vi "Robot Main.vi"() -> ()   [LabVIEW 2015]
doc: "This VI implements the framework and scheduler for your robotics program. It should not be necessary to modify the framework. You are expected to add your code to the VIs called from Robot Main - the ones located in the Team Code folder within the project."
uses:
  <vilib>/Rock Robotics/WPI/Camera/WPI_CameraImageSize.ctl
  <vilib>/Rock Robotics/WPI/Relay/WPI_RelayValue.ctl
  Robot Global Data.vi
  <vilib>/Rock Robotics/WPI/Utilities/WPI_GetSetVariantRefNum.vi
  <vilib>/Rock Robotics/WPI/Solenoid/Deprecated/WPI_SolenoidSetBool.vi
panel:
  in  "Image Size":T1=enum."320x240"
  in  "Enable Vision":bool
  in  "Finish":bool
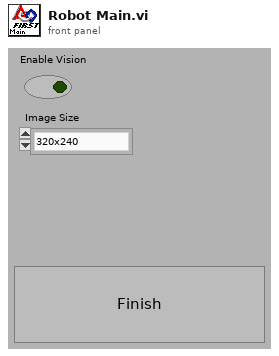
[diagram p1: front panel]
types:
  T1 = typedef "WPI_CameraImageSize.ctl" = enum16{"640x480", "320x240", "160x120", "Custom"}
  T2 = typedef "WPI_RelayValue.ctl" = enum16{"Off", "On", "Forward", "Reverse"}
  T3 = typedef "WPI_DriverStationDerivedRobotMode.ctl" = enum16{"Init", "Execute", "Stop"}
  T4 = typedef "WPI_DriverStationRobotMode2.ctl" = enum16{"Autonomous Disabled", "Autonomous Enabled", "Teleop Disabled", "Teleop Enabled", "Disconnected", "Finish", "Test Disabled", "Test Enabled", "Emergency Stopped"}
  T5 = typedef "WPI_JoystickDevRef.ctl" = cluster{"Device":T6}
  T6 = typedef "WPI_JoystickDeviceEnum.ctl" = enum16{"USB 0", "USB 1", "USB 2", "USB 3", "USB 4", "USB 5"}
  T7 = typedef "WPI_CompressorDevRef.ctl" = cluster{"DevStatus":errorcluster, "Pneumatics Control Module":u8}
  T8 = typedef "WPI_SwitchDevRef.ctl" = cluster{"DevStatus":errorcluster, "DIO Channel":T9, "CntIndex":T10, "Normally Closed":bool}
  T9 = typedef "FPGA_DIOChannel.ctl" = enum8{"DIO 0", "DIO 1", "DIO 2", "DIO 3", "DIO 4", "DIO 5", "DIO 6", "DIO 7", "DIO 8", "DIO 9", "DIO MXP 0", "DIO MXP 1", "DIO MXP 2", "DIO MXP 3", "DIO MXP 4", "DIO MXP 5", "DIO MXP 6", "DIO MXP 7", "DIO MXP 8", "DIO MXP 9", "DIO MXP 10", "DIO MXP 11", "DIO MXP 12", "DIO MXP 13", "DIO MXP 14", "DIO MXP 15", "Invalid"}
  T10 = typedef "FPGA_CounterCtrSystemIndex.ctl" = enum8{"Ctr 0", "Ctr 1", "Ctr 2", "Ctr 3", "Ctr 4", "Ctr 5", "Ctr 6", "Ctr 7", "Invalid"}
  T11 = typedef "WPI_SolenoidDevRef.ctl" = cluster{"DevStatus":errorcluster, "Pneumatics Control Module":u8, "Forward Solenoid Channel":T12, "Reverse Solenoid Channel":T12}
  T12 = typedef "WPI_SolenoidChannel.ctl" = enum8{"Solenoid 0", "Solenoid 1", "Solenoid 2", "Solenoid 3", "Solenoid 4", "Solenoid 5", "Solenoid 6", "Solenoid 7", "Invalid"}
  T13 = typedef "WPI_MotorControlDeviceRef.ctl" = cluster{"DeviceStatus":errorcluster, "Type":T14, "PWM":cluster{"PWM Channel":T15, "DeadBand":T16}, "CAN":cluster{"Device Number":u8, "Control Mode":T17, "Semaphore":T18, "Max Vout":dbl, "TalonSRX Control Mode":T19}, "Invert":bool}
  T14 = typedef "WPI_MotorControlType.ctl" = enum16{"PWM", "CAN", "CANTalonSRX"}
  T15 = typedef "FPGA_DIOPWMChannel.ctl" = enum8{"PWM 0", "PWM 1", "PWM 2", "PWM 3", "PWM 4", "PWM 5", "PWM 6", "PWM 7", "PWM 8", "PWM 9", "PWM MXP 0", "PWM MXP 1", "PWM MXP 2", "PWM MXP 3", "PWM MXP 4", "PWM MXP 5", "PWM MXP 6", "PWM MXP 7", "PWM MXP 8", "PWM MXP 9", "Invalid"}
  T16 = typedef "WPI_PWMDeadband.ctl" = cluster{"Name":string, "maxPositivePwm":i32, "minPositivePwm":i32, "centerPwm":i32, "maxNegativePwm":i32, "minNegativePwm":i32, "angularRange":u16}
  T17 = typedef "WPI_CANJaguar_ControlMode.ctl" = enum8{"Percent VBus", "Current", "Speed", "Position", "Voltage"}
  T18 = typedef "Semaphore RefNum" = refnum<k1>
  T19 = typedef "WPI_CANTalonSRX_APIControlMode.ctl" = enum8{"Percent VBus", "Speed", "Position", "Slave", "Unchanged / Invalid", "Voltage Compensation", "Current", "Motion Profile"}
  T20 = typedef "WPI_RelayDevRef.ctl" = cluster{"DevStatus":errorcluster, "Relay Channel":T21, "Relay Direction":T22}
  T21 = typedef "FPGA_DIORelayChannel.ctl" = enum8{"Relay 0", "Relay 1", "Relay 2", "Relay 3", "Invalid"}
  T22 = typedef "WPI_RelayDirection.ctl" = enum16{"Both directions", "Forward only", "Reverse only"}
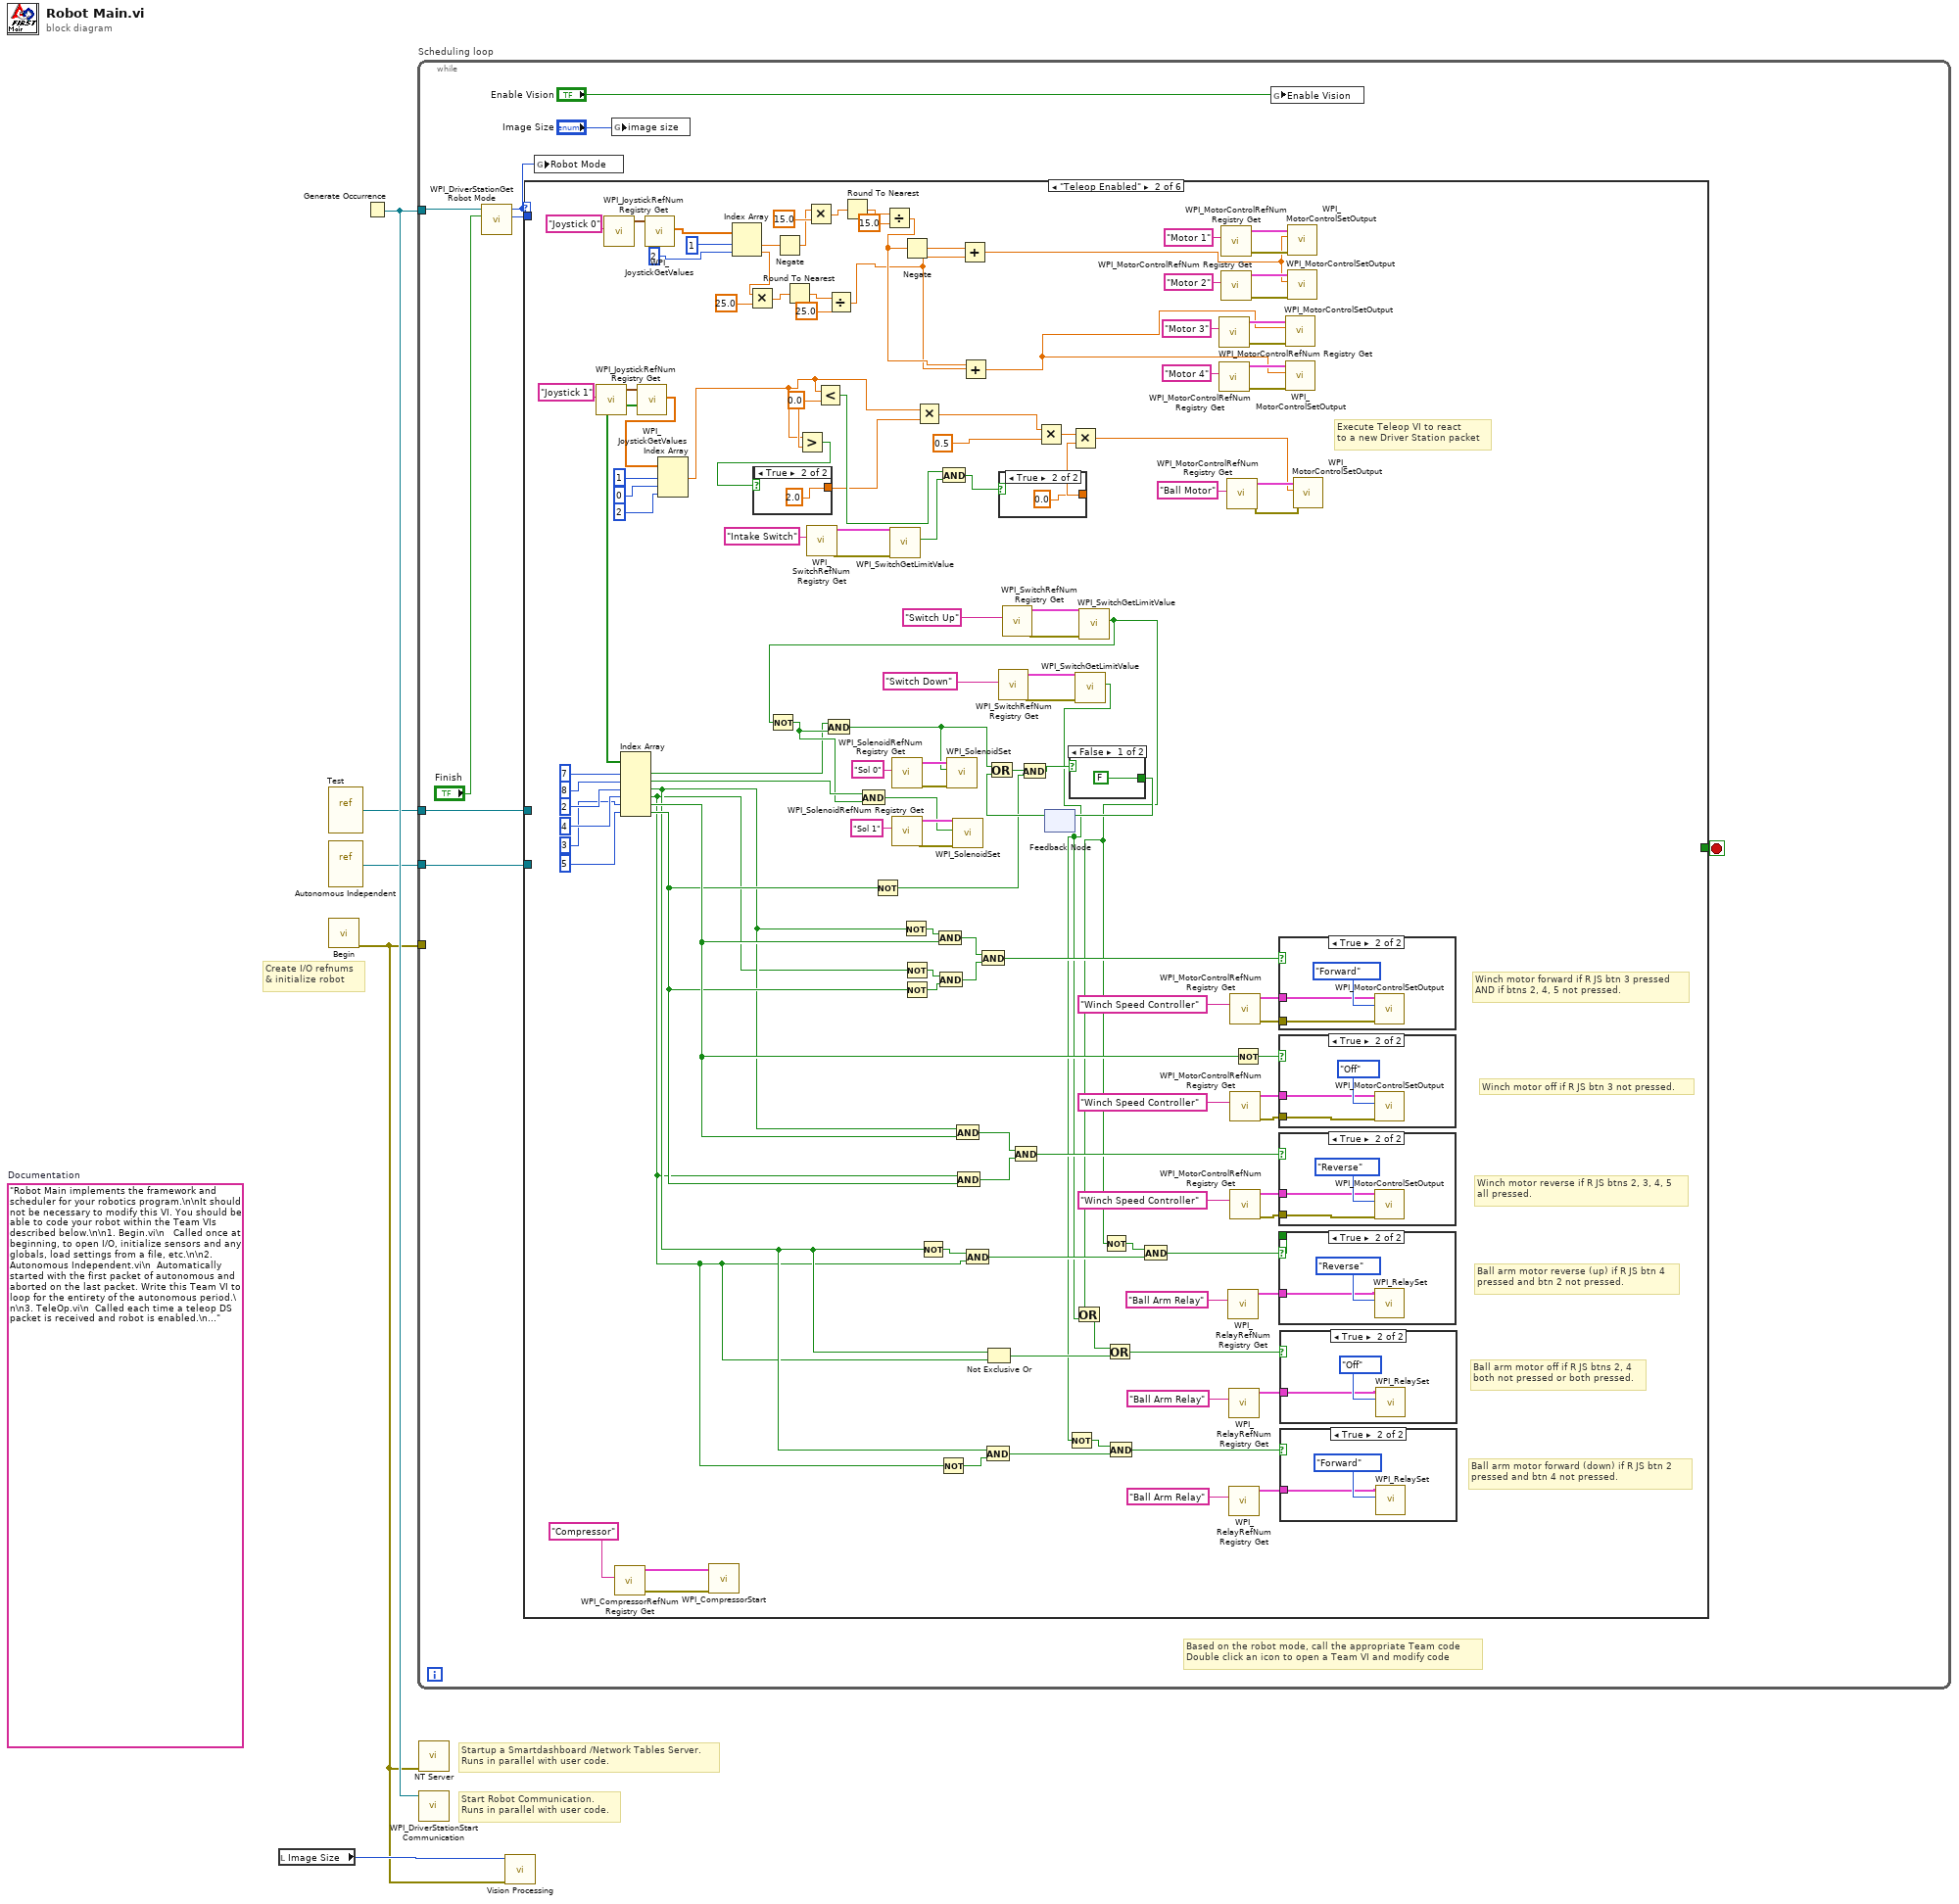
[diagram p0: block diagram]
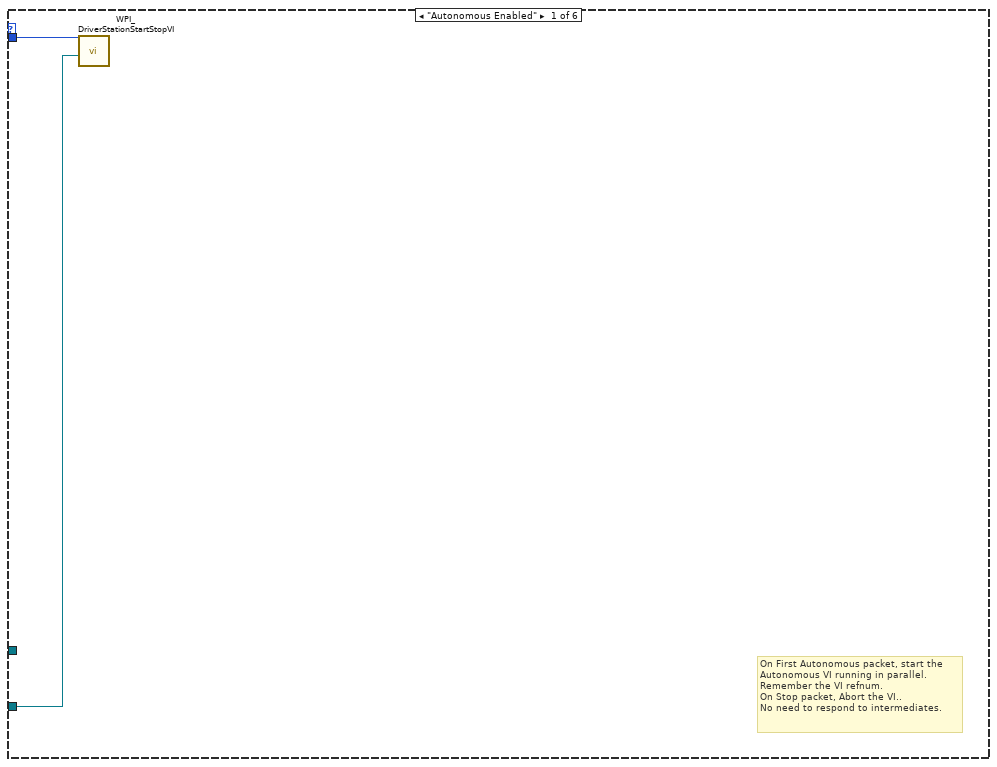
[diagram p2: hidden frame]
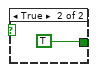
[diagram p9: hidden frame]
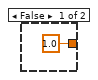
[diagram p10: hidden frame]
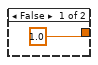
[diagram p11: hidden frame]
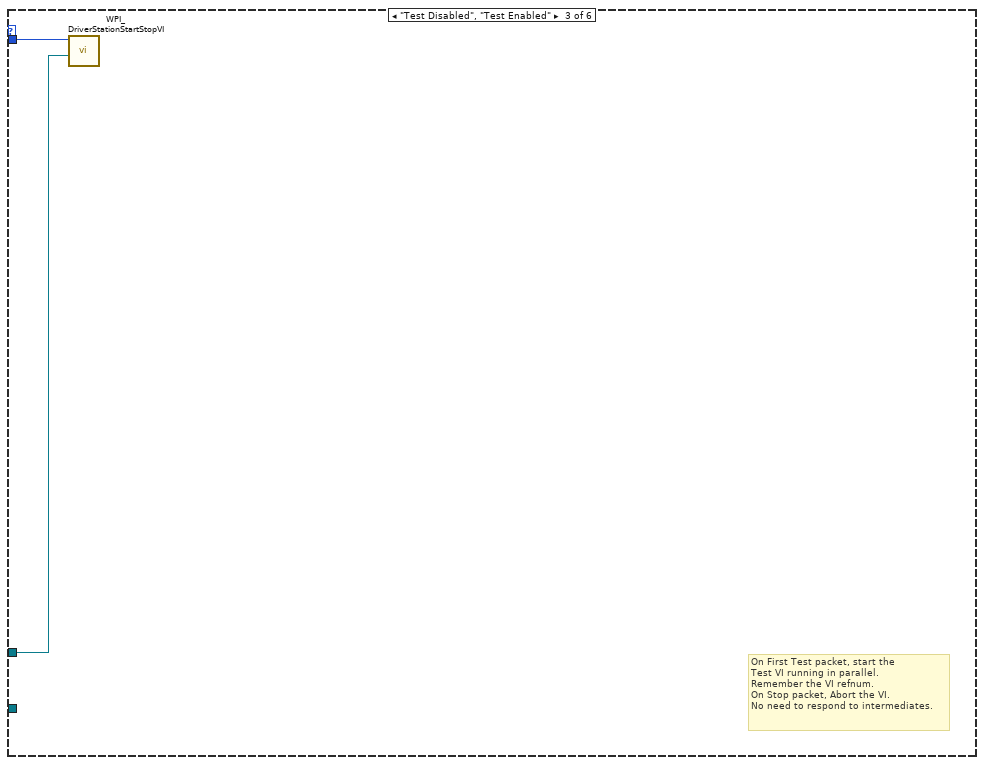
[diagram p12: hidden frame]
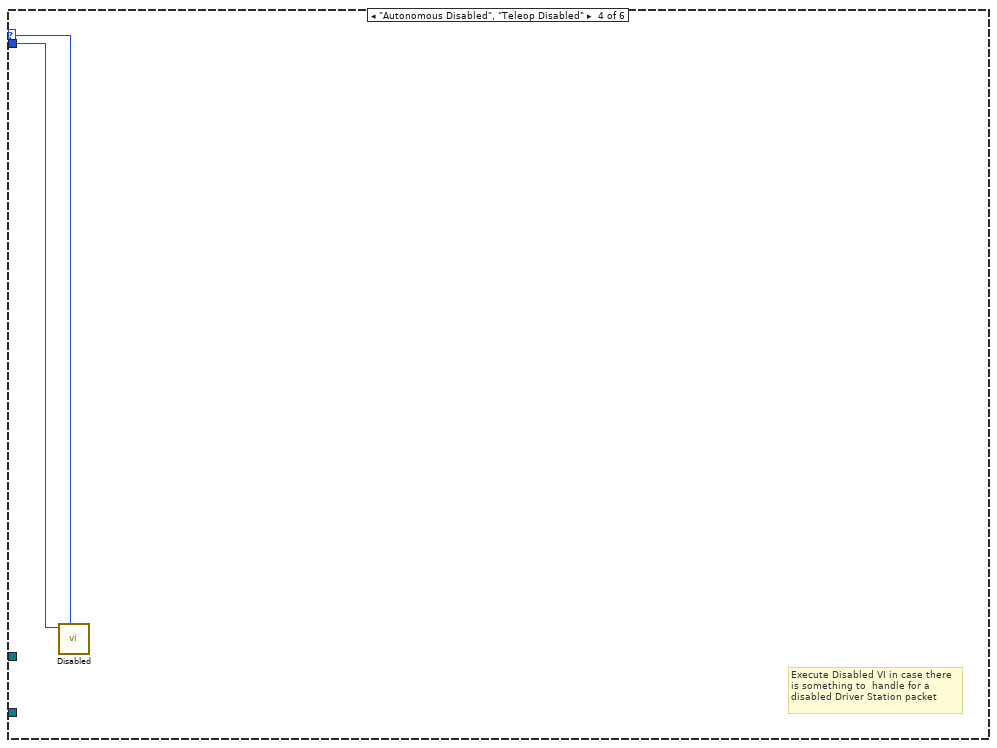
[diagram p13: hidden frame]
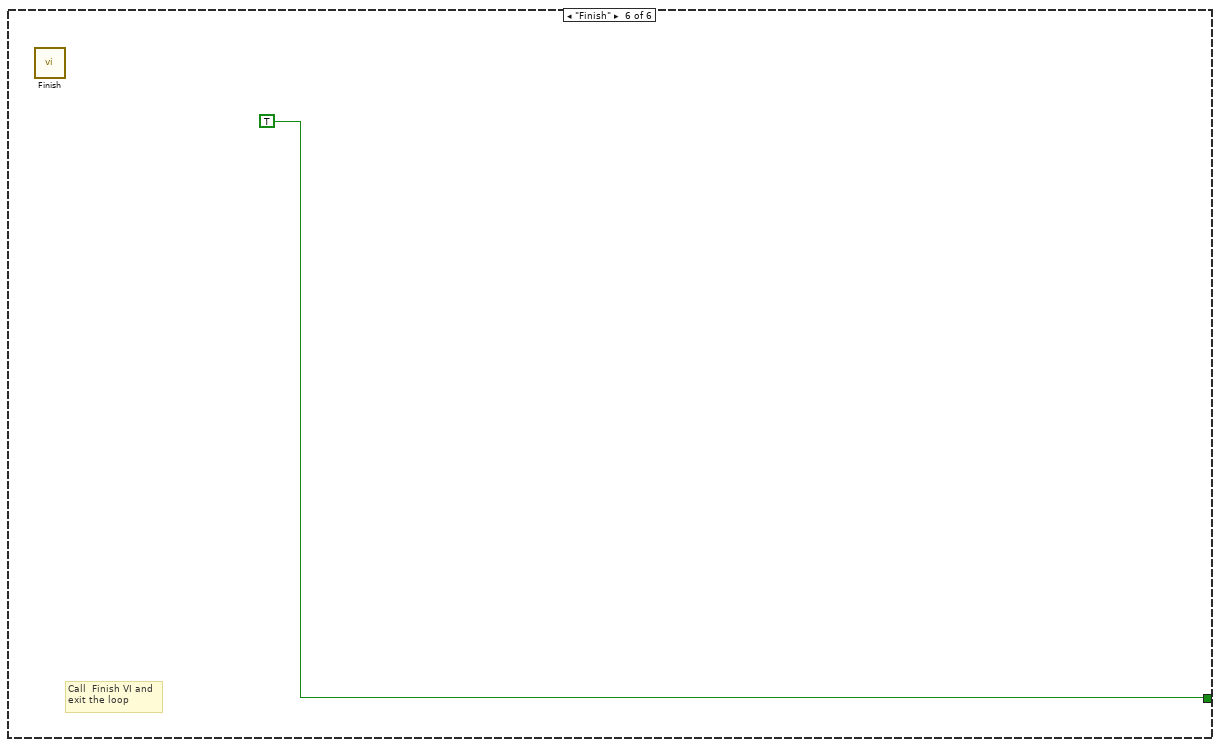
[diagram p15: hidden frame]
diagram:
  (unwired) "Robot Main implements the framework and scheduler for your robotics program.\n\nIt should not be necessary to modify this VI. You should be able to code your robot within the Team VIs described below.\n\n1. Begin.vi\n   Called once at beginning, to open I/O, initialize sensors and any globals, load settings from a file, etc.\n\n2. Autonomous Independent.vi\n  Automatically started with the first packet of autonomous and aborted on the last packet. Write this Team VI to loop for the entirety of the autonomous period.\n\n3. TeleOp.vi\n  Called each time a teleop DS packet is received and robot is enabled.\n\n4. Disabled.vi\n  Called each time a packet is received and the robot is disabled.\n\n5. Test.vi\n  Called Automatically started with the first test packet and aborted on the last. Modify this VI to carry out robot and sensor validation tests.\n\n6. Vision.vi\n  A parallel loop that acquires and processes camera images.\n\n7. PeriodicTasks.vi\n  Parallel loops running at user-defined rates.\n\n8. Finish.vi\n  Called before exiting, so you can save data, clean up I/O, etc.\n"  # Documentation
  # "Startup a Smartdashboard /Network Tables Server.\nRuns in parallel with user code."
  # "Create I/O refnums\n& initialize robot"
  # "Start Robot Communication.\nRuns in parallel with user code."
  n1 = local read "Image Size"() -> (w2:T1)
  n2 = vi-ref "Test.vi"() -> (w3:refnum<vi>)
  n3 = vi-ref "Autonomous Independent.vi"() -> (w4:refnum<vi>)
  n4 = call "Begin.vi"() -> ("error out"=w1:errorcluster)  [unwired: 2 in, 9 out]
  n5 = Generate Occurrence() -> (w5:refnum<k4>)
  n6 = while "Scheduling loop" {
    tunnel: w5 -> [w13]
    tunnel: w1 -> [_]
    tunnel: w4 -> [w9]
    tunnel: w3 -> [w7]
    stop <- w11 stop-if-true
    # "Based on the robot mode, call the appropriate Team code\nDouble click an icon to open a Team VI and modify code"
    n7 = call <vilib>:"WPI_DriverStationGet Robot Mode.vi"("Finish"="Finish", "DS Occurrence"=w13) -> ("Call Context"=w14:T3, "Robot Mode"=w6:T4)  [unwired: 8 out]
    n8 = case shown="\"Teleop Enabled\"" w6 {
      selector: w6 -> [_ _ _ w172 _ _]
      tunnel: w14 -> [w16 _ w171 w173 _ _]
      tunnel: [_ _ _ _ _ TRUE] -> w11
      tunnel: w9 -> [w15 _ _ _ _ _]
      tunnel: w7 -> [_ _ w170 _ _ _]
      frame "Autonomous Enabled" {
        # "On First Autonomous packet, start the\nAutonomous VI running in parallel.\nRemember the VI refnum.\nOn Stop packet, Abort the VI..\nNo need to respond to intermediates."
        n9 = call <vilib>:"WPI_DriverStationStartStopVI.vi"("VI in"=w15, "Call Context"=w16) -> ()  [unwired: 10 in]
      }
      frame "Teleop Enabled" {
        w106 = 0.0 ("y")
        # "Ball arm motor forward (down) if R JS btn 2\npressed and btn 4 not pressed."
        # "Ball arm motor off if R JS btns 2, 4\nboth not pressed or both pressed."
        # "Ball arm motor reverse (up) if R JS btn 4\npressed and btn 2 not pressed."
        # "Winch motor reverse if R JS btns 2, 3, 4, 5 \nall pressed."
        # "Winch motor off if R JS btn 3 not pressed."
        # "Winch motor forward if R JS btn 3 pressed\nAND if btns 2, 4, 5 not pressed."
        # "Execute Teleop VI to react\nto a new Driver Station packet"
        n10 = call <vilib>:"WPI_JoystickRefNum Registry Get.vi"("refnum name"="Joystick 1") -> ("JoystickDevRef"=w101:T5)  [unwired: 9 in, 1 out]
        n11 = call <vilib>:"WPI_JoystickRefNum Registry Get.vi"("refnum name"="Joystick 0") -> ("JoystickDevRef"=w147:T5)  [unwired: 9 in, 1 out]
        n12 = call <vilib>:"WPI_CompressorRefNum Registry Get.vi"("refnum name"="Compressor") -> ("error out"=w118:errorcluster, "CompressorDevRef"=w119:T7)  [unwired: 9 in]
        n13 = call <vilib>:"WPI_JoystickGetValues.vi"("JoystickDevRef"=w101) -> ("Buttons"=w99:bool[], "Axes"=w100:dbl[])  [unwired: 6 in, 3 out]
        n14 = Index Array(array=w99, index #1=7 ("index"), index #2=8 ("index"), index #3=2 ("index"), index #4=4 ("index"), index #5=3 ("index"), index #6=5 ("index")) -> (element #1=w83:bool, element #2=w87:bool, element #3=w50:bool, element #4=w49:bool, element #5=w62:bool, element #6=w57:bool)
        n15 = call <vilib>:"WPI_JoystickGetValues.vi"("JoystickDevRef"=w147) -> ("Axes"=w145:dbl[])  [unwired: 6 in, 4 out]
        n16 = Index Array(array=w100, index #1=1 ("index"), index #2=0 ("index"), index #3=2 ("index")) -> (element #1=w96:dbl)  [unwired: 2 out]
        n17 = call <vilib>:"WPI_CompressorStart.vi"("error in (no error)"=w118, "CompressorDevRef"=w119) -> ()  [unwired: 8 in, 2 out]
        n18 = Index Array(array=w145, index #1=1 ("index"), index #2=2 ("index")) -> (element #1=w23:dbl, element #2=w25:dbl)
        n19 = Multiply(x=w25, y=25.0) -> (x*y=w34:dbl)
        n20 = Negate(x=w23) -> (-x=w24:dbl)
        n21 = Round To Nearest(number=w34) -> (nearest integer value=w33:dbl)
        n22 = Greater?(x=w96, y=w106) -> (0:w105:bool)
        n23 = case shown="True" w105 {
          tunnel: [1.0 2.0] -> w103
          frame False {
          }
          frame True {
          }
        }
        n24 = Multiply(x=w24, y=15.0) -> (x*y=w31:dbl)
        n25 = call <vilib>:"WPI_SwitchRefNum Registry Get.vi"("refnum name"="Intake Switch") -> ("error out"=w114:errorcluster, "SwitchDevRef"=w115:T8)  [unwired: 9 in]
        n26 = Less?(x=w96, y=w106) -> (x < y?=w108:bool)
        n27 = Divide(x=w33, y=25.0) -> (x/y=w22:dbl)
        n28 = Round To Nearest(number=w31) -> (nearest integer value=w32:dbl)
        n29 = Not(x=w57) -> (.not. x?=w80:bool)
        n30 = Divide(x=w32, y=15.0) -> (x/y=w26:dbl)
        n31 = call <vilib>:"WPI_SwitchGetLimitValue.vi"("error in (no error)"=w114, "SwitchDevRef"=w115) -> ("Switch Pressed"=w109:bool)  [unwired: 7 in, 2 out]
        n32 = call <vilib>:"WPI_SolenoidRefNum Registry Get.vi"("refnum name"="Sol 0") -> ("error out"=w124:errorcluster, "SolenoidDevRef"=w125:T11)  [unwired: 9 in]
        n33 = call <vilib>:"WPI_SolenoidRefNum Registry Get.vi"("refnum name"="Sol 1") -> ("error out"=w122:errorcluster, "SolenoidDevRef"=w123:T11)  [unwired: 9 in]
        n34 = Not(x=w50) -> (.not. x?=w68:bool)
        n35 = Negate(x=w26) -> (-x=w35:dbl)
        n36 = Not(x=w49) -> (.not. x?=w67:bool)
        n37 = Not(x=w57) -> (.not. x?=w66:bool)
        n38 = Multiply(x=w96, y=w103) -> (x*y=w104:dbl)
        n39 = Not(x=w50) -> (.not. x?=w52:bool)
        n40 = And(x=w68, y=w62) -> (x .and. y?=w65:bool)
        n41 = And(x=w67, y=w66) -> (x .and. y?=w64:bool)
        n42 = Not(x=w49) -> (.not. x?=w51:bool)
        n43 = And(x=w108, y=w109) -> (x .and. y?=w107:bool)
        n44 = And(x=w50, y=w62) -> (x .and. y?=w72:bool)
        n45 = And(x=w49, y=w57) -> (x .and. y?=w71:bool)
        n46 = Add(x=w35, y=w22) -> (x+y=w131:dbl)
        n47 = Add(x=w26, y=w22) -> (x+y=w132:dbl)
        n48 = And(x=w52, y=w49) -> (x .and. y?=w44:bool)
        n49 = And(x=w65, y=w64) -> (x .and. y?=w63:bool)
        n50 = And(x=w50, y=w51) -> (x .and. y?=w48:bool)
        n51 = Not Exclusive Or(1:w49, 2:w50) -> (0:w42:bool)
        n52 = case shown="True" w107 {
          tunnel: [1.0 0.0] -> w110
          frame False {
          }
          frame True {
          }
        }
        n53 = call <vilib>:"WPI_SwitchRefNum Registry Get.vi"("refnum name"="Switch Down") -> ("error out"=w93:errorcluster, "SwitchDevRef"=w92:T8)  [unwired: 9 in]
        n54 = call <vilib>:"WPI_SwitchRefNum Registry Get.vi"("refnum name"="Switch Up") -> ("error out"=w90:errorcluster, "SwitchDevRef"=w91:T8)  [unwired: 9 in]
        n55 = And(x=w72, y=w71) -> (x .and. y?=w70:bool)
        n56 = Multiply(x=w104, y=0.5) -> (x*y=w112:dbl)
        n57 = feedback #1() -> (w85:bool)  [unwired: 1 in]
        n58 = Multiply(x=w112, y=w110) -> (x*y=w111:dbl)
        n59 = call <vilib>:"WPI_SwitchGetLimitValue.vi"("error in (no error)"=w93, "SwitchDevRef"=w92) -> ("Switch Pressed"=w38:bool)  [unwired: 7 in, 2 out]
        n60 = Not(x=w38) -> (.not. x?=w46:bool)
        n61 = call <vilib>:"WPI_SwitchGetLimitValue.vi"("error in (no error)"=w90, "SwitchDevRef"=w91) -> ("Switch Pressed"=w39:bool)  [unwired: 7 in, 2 out]
        n62 = Not(x=w39) -> (.not. x?=w86:bool)
        n63 = And(x=w83, y=w86) -> (x .and. y?=w79:bool)
        n64 = And(x=w87, y=w86) -> (x .and. y?=w88:bool)
        n65 = call-poly <vilib>:"WPI_SolenoidSet.vi"("error in (no error)"=w124, "Value"=w79, "SolenoidDevRef"=w125) -> ()  [unwired: 7 in, 2 out]
        n66 = call-poly <vilib>:"WPI_SolenoidSet.vi"("error in (no error)"=w122, "Value"=w88, "SolenoidDevRef"=w123) -> ()  [unwired: 7 in, 2 out]
        n67 = Or(x=w79, y=w85) -> (x .or. y?=w81:bool)
        n68 = And(x=w81, y=w80) -> (x .and. y?=w82:bool)
        n69 = case shown="False" w82 {
          tunnel: [FALSE TRUE] -> w84
          frame False {
          }
          frame True {
          }
        }
        n70 = feedback-in #1(w84) -> ()
        n71 = Or(x=w39, y=w38) -> (x .or. y?=w41:bool)
        n72 = Not(x=w39) -> (.not. x?=w45:bool)
        n73 = Or(x=w41, y=w42) -> (x .or. y?=w40:bool)
        n74 = And(x=w46, y=w48) -> (x .and. y?=w47:bool)
        n75 = And(x=w45, y=w44) -> (x .and. y?=w43:bool)
        n76 = call <vilib>:"WPI_MotorControlRefNum Registry Get.vi"("refnum name"="Motor 3") -> ("error out"=w134:errorcluster, "MotorControlDevRef"=w133:T13)  [unwired: 9 in]
        n77 = call <vilib>:"WPI_MotorControlRefNum Registry Get.vi"("refnum name"="Motor 4") -> ("error out"=w137:errorcluster, "MotorControlDevRef"=w138:T13)  [unwired: 9 in]
        n78 = call <vilib>:"WPI_MotorControlRefNum Registry Get.vi"("refnum name"="Motor 1") -> ("error out"=w143:errorcluster, "MotorControlDevRef"=w144:T13)  [unwired: 9 in]
        n79 = call <vilib>:"WPI_MotorControlRefNum Registry Get.vi"("refnum name"="Motor 2") -> ("error out"=w140:errorcluster, "MotorControlDevRef"=w139:T13)  [unwired: 9 in]
        n80 = call <vilib>:"WPI_MotorControlRefNum Registry Get.vi"("refnum name"="Ball Motor") -> ("error out"=w129:errorcluster, "MotorControlDevRef"=w128:T13)  [unwired: 9 in]
        n81 = call <vilib>:"WPI_RelayRefNum Registry Get.vi"("refnum name"="Ball Arm Relay") -> ("RelayDevRef"=w75:T20)  [unwired: 9 in, 1 out]
        n82 = call <vilib>:"WPI_RelayRefNum Registry Get.vi"("refnum name"="Ball Arm Relay") -> ("RelayDevRef"=w56:T20)  [unwired: 9 in, 1 out]
        n83 = call <vilib>:"WPI_RelayRefNum Registry Get.vi"("refnum name"="Ball Arm Relay") -> ("RelayDevRef"=w54:T20)  [unwired: 9 in, 1 out]
        n84 = call <vilib>:"WPI_MotorControlRefNum Registry Get.vi"("refnum name"="Winch Speed Controller") -> ("error out"=w73:errorcluster, "MotorControlDevRef"=w17:T13)  [unwired: 9 in]
        n85 = call <vilib>:"WPI_MotorControlRefNum Registry Get.vi"("refnum name"="Winch Speed Controller") -> ("error out"=w18:errorcluster, "MotorControlDevRef"=w19:T13)  [unwired: 9 in]
        n86 = call <vilib>:"WPI_MotorControlRefNum Registry Get.vi"("refnum name"="Winch Speed Controller") -> ("error out"=w21:errorcluster, "MotorControlDevRef"=w20:T13)  [unwired: 9 in]
        n87 = Not(x=w62) -> (.not. x?=w69:bool)
        n88 = case shown="True" w63 {
          tunnel: w73 -> [_ w162]
          tunnel: w17 -> [_ w161]
          frame False {
          }
          frame True {
            n89 = call <vilib>:"WPI_MotorControlSetOutput.vi"("error in (no error)"=w162, "Output"=WPI_RelayValue."Forward" ("RelayValue"), "MotorControlDevRef"=w161) -> ()  [unwired: 6 in, 3 out]
          }
        }
        n90 = case shown="True" w69 {
          tunnel: w19 -> [_ w159]
          tunnel: w18 -> [_ w158]
          frame False {
          }
          frame True {
            n91 = call <vilib>:"WPI_MotorControlSetOutput.vi"("error in (no error)"=w158, "Output"=WPI_RelayValue."Off" ("RelayValue"), "MotorControlDevRef"=w159) -> ()  [unwired: 6 in, 3 out]
          }
        }
        n92 = case shown="True" w70 {
          tunnel: w21 -> [_ w156]
          tunnel: w20 -> [_ w155]
          frame False {
          }
          frame True {
            n93 = call <vilib>:"WPI_MotorControlSetOutput.vi"("error in (no error)"=w156, "Output"=WPI_RelayValue."Reverse" ("RelayValue"), "MotorControlDevRef"=w155) -> ()  [unwired: 6 in, 3 out]
          }
        }
        n94 = case shown="True" w43 {
          selector: w43 -> [_ w152]
          tunnel: w75 -> [_ w153]
          tunnel: [_ w152] -> _
          frame False {
          }
          frame True {
            n95 = call <vilib>:"WPI_RelaySet.vi"("RelayValue"=WPI_RelayValue."Reverse", "RelayDevRef"=w153) -> ()  [unwired: 8 in, 2 out]
          }
        }
        n96 = case shown="True" w40 {
          tunnel: w56 -> [_ w150]
          frame False {
          }
          frame True {
            n97 = call <vilib>:"WPI_RelaySet.vi"("RelayValue"=WPI_RelayValue."Off", "RelayDevRef"=w150) -> ()  [unwired: 8 in, 2 out]
          }
        }
        n98 = case shown="True" w47 {
          tunnel: w54 -> [_ w148]
          frame False {
          }
          frame True {
            n99 = call <vilib>:"WPI_RelaySet.vi"("RelayValue"=WPI_RelayValue."Forward", "RelayDevRef"=w148) -> ()  [unwired: 8 in, 2 out]
          }
        }
        n100 = call <vilib>:"WPI_MotorControlSetOutput.vi"("error in (no error)"=w134, "Output"=w132, "MotorControlDevRef"=w133) -> ()  [unwired: 6 in, 3 out]
        n101 = call <vilib>:"WPI_MotorControlSetOutput.vi"("error in (no error)"=w137, "Output"=w132, "MotorControlDevRef"=w138) -> ()  [unwired: 6 in, 3 out]
        n102 = call <vilib>:"WPI_MotorControlSetOutput.vi"("error in (no error)"=w143, "Output"=w131, "MotorControlDevRef"=w144) -> ()  [unwired: 6 in, 3 out]
        n103 = call <vilib>:"WPI_MotorControlSetOutput.vi"("error in (no error)"=w140, "Output"=w131, "MotorControlDevRef"=w139) -> ()  [unwired: 6 in, 3 out]
        n104 = call <vilib>:"WPI_MotorControlSetOutput.vi"("error in (no error)"=w129, "Output"=w111, "MotorControlDevRef"=w128) -> ()  [unwired: 6 in, 3 out]
      }
      frame "Test Disabled", "Test Enabled" {
        # "On First Test packet, start the\nTest VI running in parallel.\nRemember the VI refnum.\nOn Stop packet, Abort the VI.\nNo need to respond to intermediates."
        n105 = call <vilib>:"WPI_DriverStationStartStopVI.vi"("VI in"=w170, "Call Context"=w171) -> ()  [unwired: 10 in]
      }
      frame "Autonomous Disabled", "Teleop Disabled" {
        # "Execute Disabled VI in case there\nis something to  handle for a\ndisabled Driver Station packet"
        n106 = call "Disabled.vi"("Robot Mode"=w172, "Call Context"=w173) -> ()  [unwired: 2 in, 8 out]
      }
      frame "Disconnected", Default {
        # "Driver Station packet didn't arrive.\nPossibly useful for diagnostics"
      }
      frame "Finish" {
        # "Call  Finish VI and\nexit the loop"
        n107 = call "Finish.vi"() -> ()  [unwired: 1 in, 7 out]
      }
    }
    n108 = global write "Robot Global Data.vi" "Robot Mode"(w6) -> ()
    n109 = global write "Robot Global Data.vi" "image size"("Image Size") -> ()
    n110 = global write "Robot Global Data.vi" "Enable Vision"("Enable Vision") -> ()
  }
  n111 = call <vilib>:"NT Server.vi"("error in (no error)"=w1) -> ()  [unwired: 11 in]
  n112 = call <vilib>:"WPI_DriverStationStart Communication.vi"("occurrence"=w5) -> ()  [unwired: 1 in, 10 out]
  n113 = call "Vision Processing.vi"("error in (no error)"=w1, "Image Size"=w2) -> ()  [unwired: 6 out]
